vi "Excel Try Opening Excel Again.vi"(4 "machine name (empty)":string, 6 "display alerts? (F)":bool, 8 "error in (no error)":errorcluster, 9 "window state (normal)":T1(ring), 10 "Excel._Application in":refnum<k7>) -> (0 "error out":errorcluster, 2 "Excel._Application out":refnum<k7>)   [LabVIEW 2010, in "NI_ReportGenerationToolkit.lvlib"]
uses:
  <vilib>/addons/_office/NI_ReportGenerationToolkit.lvlib
panel:
  in  "Excel._Application":refnum<k7>
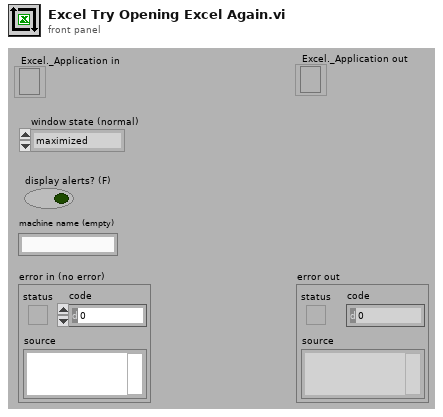
[diagram p1: front panel]
types:
  T1 = enum16{"maximized", "minimized", "normal", "no change"}
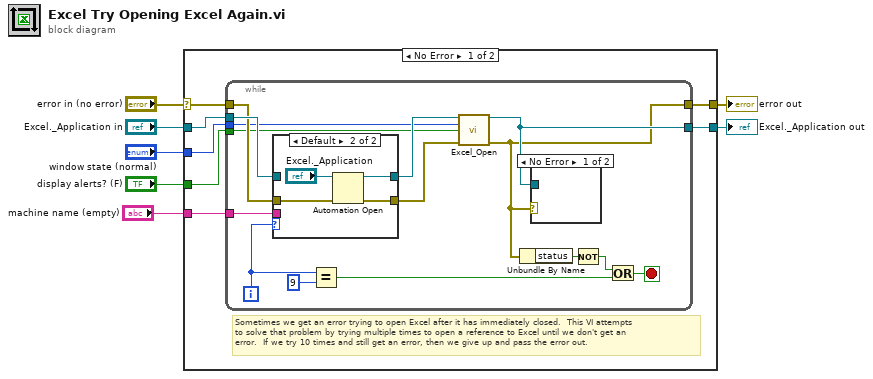
[diagram p0: block diagram]
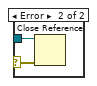
[diagram p2: hidden frame]
diagram:
  n1 = case shown="No Error" "error in (no error)" {
    selector: "error in (no error)" -> [w9 w38]
    tunnel: [w14 w39] -> w7
    tunnel: "display alerts? (F)" -> [w13 _]
    tunnel: "window state (normal)" -> [w12 _]
    tunnel: "Excel._Application in" -> [w11 w39]
    tunnel: [w8 w38] -> w3
    tunnel: "machine name (empty)" -> [w10 _]
    frame No Error {
      # "Sometimes we get an error trying to open Excel after it has immediately closed.  This VI attempts\nto solve that problem by trying multiple times to open a reference to Excel until we don't get an\nerror.  If we try 10 times and still get an error, then we give up and pass the error out."
      n2 = while {
        tunnel: w13 -> [w18]
        tunnel: w12 -> [w19]
        tunnel: w9 -> [w28]
        tunnel: w11 -> [w29]
        tunnel: [w17] -> w14
        tunnel: w10 -> [w27]
        tunnel: [w15] -> w8
        i -> [w26]
        stop <- w21 stop-if-true
        n3 = case shown="Default" w26 {
          tunnel: w29 -> [w33 _]
          tunnel: [w33 w36] -> w20
          tunnel: w28 -> [w32 w35]
          tunnel: [w32 w34] -> w16
          tunnel: w27 -> [_ _]
          frame 0 {
          }
          frame Default {
            n4 = Automation Open(error in (no error)=w35, Automation Refnum="Excel._Application") -> (Automation Refnum=w36:refnum<k7>, error out=w34:errorcluster)  [unwired: 2 out]
          }
        }
        n5 = Equal?(x=w26, y=9) -> (x = y?=w24:bool)
        n6 = call <vilib>:"Excel_Open.vi"("excel application in"=w20, "window state"=w19, "display alerts?"=w18, "error in"=w16) -> ("excel application out"=w17:refnum<k7>, "error out"=w15:errorcluster)  [unwired: 10 out]
        n7 = Unbundle By Name(w15) -> ("status"=w22:bool)
        n8 = case shown="No Error" w15 {
          selector: w15 -> [_ w31]
          tunnel: w17 -> [_ w30]
          frame No Error {
          }
          frame Error {
            n9 = Close Reference(reference=w30, error in (no error)=w31) -> ()  [unwired: 1 out]
          }
        }
        n10 = Not(x=w22) -> (.not. x?=w23:bool)
        n11 = Or(x=w23, y=w24) -> (x .or. y?=w21:bool)
      }
    }
    frame Error {
    }
  }
  "Excel._Application out" <- w7
  "error out" <- w3
